vi "PLC断开.vi"(8 "错误输入（无错误）":errorcluster, 11 "引用":refnum<k24>) -> (0 "错误输出":errorcluster, 3 "引用输出":refnum<k24>)   [LabVIEW 2021]
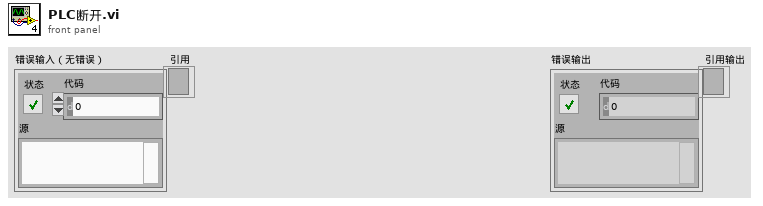
[diagram p1: front panel]
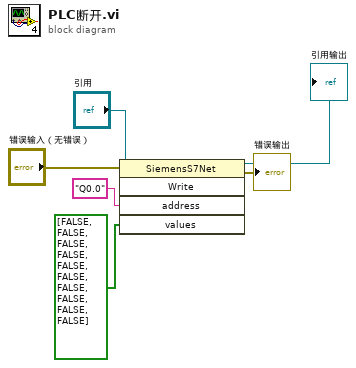
[diagram p0: block diagram]
diagram:
  n1 = invoke class="SiemensS7Net" method="Write"(reference="引用", error in="错误输入（无错误）", "address"="Q0.0", "values"=bool[] [FALSE, FALSE, FALSE, FALSE, FALSE, FALSE, FALSE, FALSE, FALSE, FALSE]) -> (reference out=→"引用输出":refnum<k24>, error out=→"错误输出":errorcluster)  [unwired: 1 in, 3 out]
